vi "RelayOpen_L.vi"(0 "datain":string[](array[string])=["备注", "负载通道", "负载地址", "延时时间", "output max", "output min", "量测类型", "待测物板号"], 5 "HW CH Number":i32=4, 7 "Setup":string) -> (4 "REPORT INDECATE":string[][](array[string])=[["微安测试", "", "", "", ""], ["微安量测", "4", "0.000", "0.1", "NG"], ["微安量测", "4", "0.000", "0.1", "NG"], ["微安量测", "4", "0.000", "0.1", "NG"], ["微安量测", "4", "0.000", "0.1", "NG"]], 6 "ROW HEAD":string[](array[string]), 8 "PF":string[](array[string]), 10 "testData":string[](array[string]), 14 "数组":bool[](array[boolean]), 15 "Array":string[](array[string]))   [LabVIEW 2018]
uses:
  Subvi/Global.vi
panel:
  out "数组 2":string[](array[string])
  out "CMD 2":string
  out "测试板数":i32=4
  # "Ext.Name =Cylinder_Open;\nAddress =0;\nDelay Time =100;\nMAX.Spec =*;\nMin.Spec =*;\nTest Type =4;\nRelayH_8Bit =3,0,0,;\nRelayL_8Bit =3,0,0,;\nStandby Application =;\nStart board number =1;#"
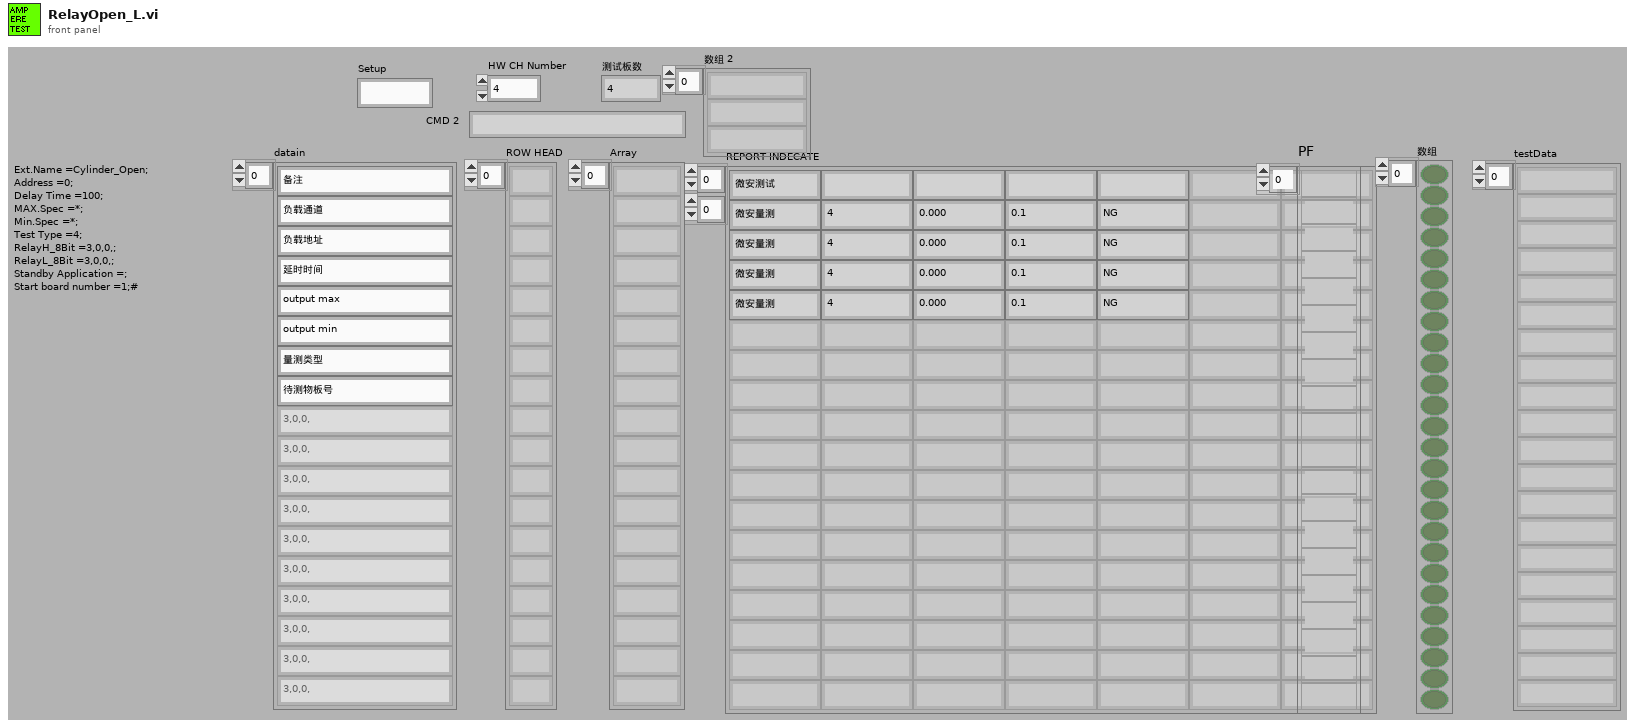
[diagram p1: front panel]
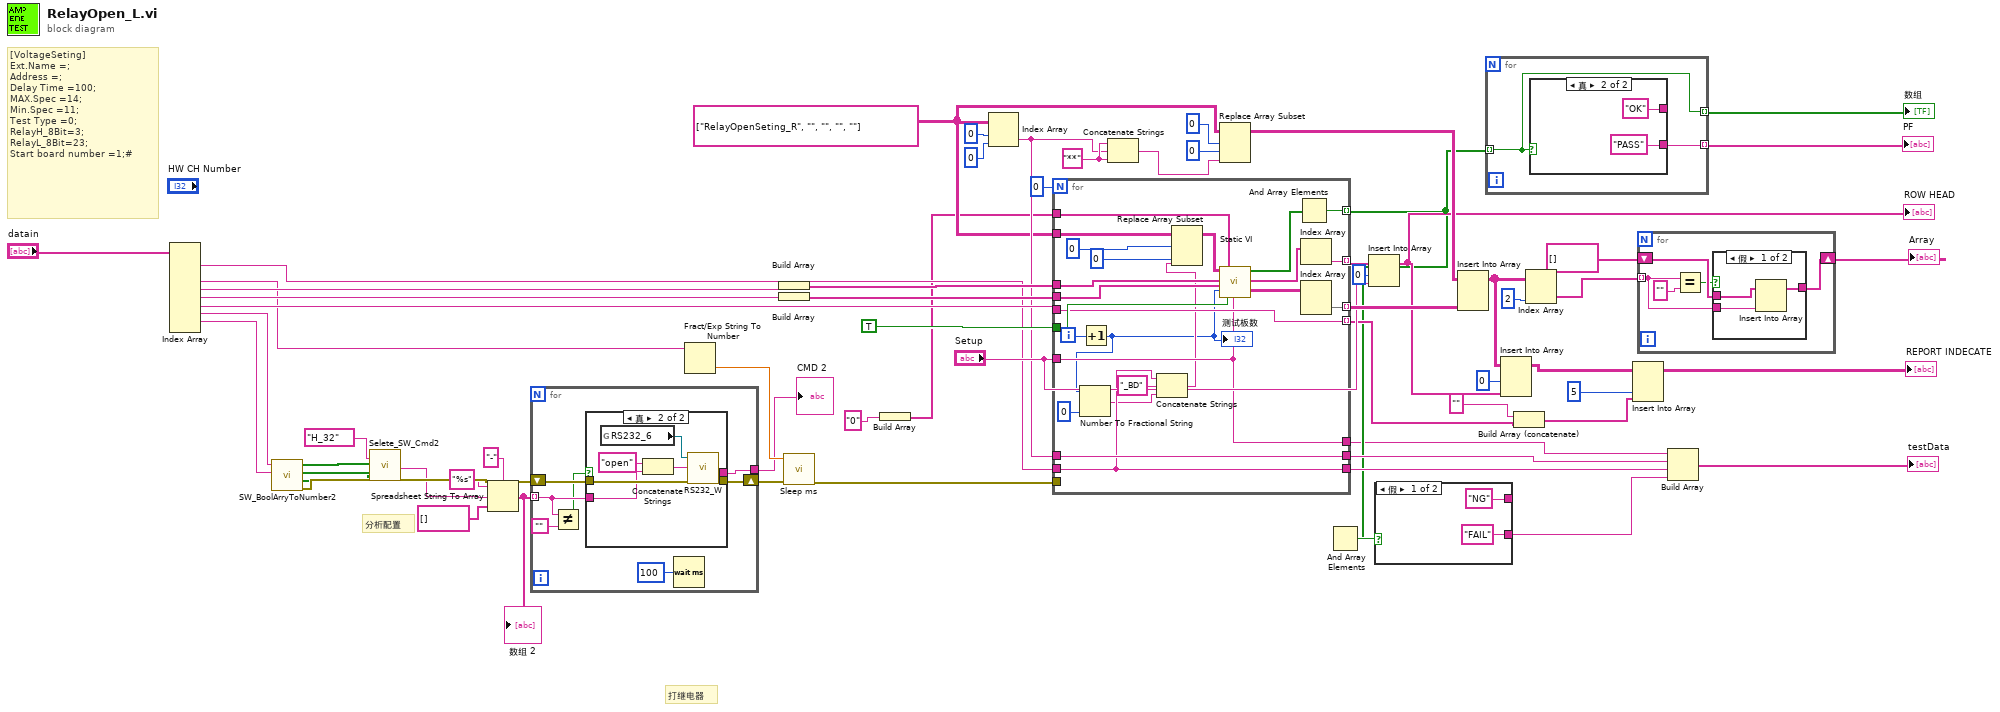
[diagram p0: block diagram]
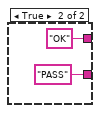
[diagram p3: hidden frame]
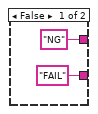
[diagram p4: hidden frame]
diagram:
  w22 = string[][] [["RelayOpenSeting_R", "", "", "", ""]]
  w56 = "**" ("字符串")
  # "分析配置"
  # "打继电器"
  # "[VoltageSeting]\nExt.Name =;\nAddress =;\nDelay Time =100;\nMAX.Spec =14;\nMin.Spec =11;\nTest Type =0;\nRelayH_8Bit=3;\nRelayL_8Bit=23;\nStart board number =1;#"
  n1 = Index Array(array="datain") -> (element #1=w23:string, element #3=w16:string, element #4=w52:string, element #5=w51:string, element #6=w39:string, element #7=w15:string, element #8=w14:string)  [unwired: 9 in, 2 out]
  n2 = call "SW_BoolArryToNumber2.vi"("L32 INUPT"=w14, "H32 INUPT"=w15) -> ("error out"=w10:errorcluster, "64 SW OUT"=w7:bool[], "L_32"=w12:bool[], "H_32"=w18:bool[])  [unwired: 6 in]
  n3 = call "Selete_SW_Cmd2.vi"("组合框"="H_32", "H_32"=w18, "L_32"=w12, "64 SW OUT"=w7, "error in (no error)"=w10) -> ("OpenStr2"=w1:string, "error out"=w9:errorcluster)  [unwired: 11 in, 2 out]
  n4 = Spreadsheet String To Array(delimiter (Tab)="-" ("分隔符(Tab)"), format string="%s" ("格式字符串"), spreadsheet string=w1, array type (2D Dbl)=string[] []) -> (array=w2:string[])
  "数组 2" <- w2
  n5 = for {
    tunnel: [w69] -> w6
    shift-right: [w70] -> w8
    shift-left: w9 -> [w71]
    tunnel: w2 -> [w67] mode=indexing
    n6 = Not Equal?(x=w67, y="") -> (x != y?=w66:bool)
    n7 = case shown="真" w66 {
      tunnel: w71 -> [w72 w79]
      tunnel: [w72 w78] -> w70
      tunnel: [_ w76] -> w69
      tunnel: w67 -> [_ w73]
      frame False {
      }
      frame True {
        n8 = global read "Global.vi" "RS232_6"() -> (w77:refnum<visa-resource-name>)
        n9 = Concatenate Strings("open", w73) -> (w75:string)
        n10 = call "RS232_W.vi"("error in (no error)"=w79, "CMD"=w75, "VISA资源名称"=w77) -> ("error out"=w78:errorcluster, "CMD 2"=w76:string)  [unwired: 6 in, 1 out]
      }
    }
    n11 = Wait (ms)(milliseconds to wait=u32 100 ("等待时间（毫秒）")) -> ()  [unwired: 1 out]
  }
  "CMD 2" <- w6
  n12 = Fract/Exp String To Number(string=w16) -> (number=w17:dbl)  [unwired: 3 in, 1 out]
  n13 = Build Array(w52) -> (w50:string[])
  n14 = Build Array(w51) -> (w49:string[])
  n15 = call "Sleep ms.vi"("error in (no error)"=w8, "等待时间（毫秒）"=w17) -> ("error out"=w13:errorcluster)  [unwired: 9 in]
  n16 = Build Array("0") -> (w19:string[])
  n17 = Index Array(array=w22, index (row)=0 ("索引 (行)"), index (col)=0 ("禁用的索引 (列)")) -> (element=w32:string)
  n18 = for {
    N: 0 -> [_]
    tunnel: w19 -> [w103]
    tunnel: w50 -> [w102]
    tunnel: w49 -> [w101]
    tunnel: "Setup" -> [w91]
    tunnel: TRUE -> [w99]
    tunnel: [w98] -> w28 mode=indexing
    tunnel: [w96] -> w45 mode=indexing
    tunnel: [w94] -> w46 mode=indexing
    tunnel: w39 -> [w93]
    tunnel: [w93] -> w35 mode=indexing
    tunnel: w32 -> [w92]
    tunnel: [w92] -> w31
    tunnel: w23 -> [w83]
    tunnel: [w83] -> w30
    tunnel: [w91] -> w25
    tunnel: w22 -> [w89]
    tunnel: w13 -> [_]
    i -> [w86]
    n19 = Increment(x=w86) -> (x+1=w80:i32)
    "测试板数" <- w80
    n20 = Number To Fractional String(number=w80, precision (6)=i16 0 ("精度(6)")) -> (F-format string=w82:string)  [unwired: 2 in]
    n21 = Concatenate Strings(w83, "_BD" ("字符串"), w82) -> (w81:string)
    n22 = Replace Array Subset(array=w89, new element=w81, index (row)=0 ("索引 (行)"), index (col)=0 ("禁用的索引 (列)")) -> (w88:string[][])
    n23 = call "Static VI.vi"("添加的数组"=w88, "Max"=w102, "Min"=w101, "板数"=w80, "INPUTSTRING"=w103, "是否为字符串对比"=w99, "SQ"=w91) -> ("P/F"=w100:bool[], "SQ out"=w97:string[], "arrauy out"=w95:string[][])  [unwired: 9 in, 1 out]
    n24 = And Array Elements(Boolean array=w100) -> (logical AND=w98:bool)
    n25 = Index Array(array=w97) -> (element=w96:string)  [unwired: 1 in]
    n26 = Index Array(array=w95) -> (element=w94:string[])  [unwired: 2 in]
  }
  n27 = Concatenate Strings(w56, w32, w56) -> (w53:string)
  n28 = Replace Array Subset(array=w22, new element=w53, index (row)=0 ("索引 (行)"), index (col)=0 ("禁用的索引 (列)")) -> (w47:string[][])
  n29 = And Array Elements(Boolean array=w28) -> (logical AND=w29:bool)
  n30 = Insert Into Array(array=w45, index=0 ("索引"), new element="Setup") -> (w41:string[])
  "ROW HEAD" <- w41
  n31 = case shown="假" w29 {
    tunnel: ["NG" "OK"] -> _
    tunnel: ["FAIL" "PASS"] -> w27
    frame False {
    }
    frame True {
    }
  }
  n32 = Insert Into Array ("数组插入")(array=w47, new element=w46) -> (w42:string[][])  [unwired: 2 in]
  n33 = for {
    tunnel: w28 -> [w108] mode=indexing
    tunnel: [w109] -> w60 mode=indexing
    tunnel: [w108] -> w24 mode=indexing
    n34 = case shown="真" w108 {
      tunnel: ["NG" "OK"] -> _
      tunnel: ["FAIL" "PASS"] -> w109
      frame False {
      }
      frame True {
      }
    }
  }
  "PF" <- w60
  "数组" <- w24
  n35 = Insert Into Array(array=w42, index (col)=0 ("禁用的索引 (列)"), new element=w41) -> (w37:string[][])  [unwired: 1 in]
  n36 = Build Array (concatenate)("" ("字符串"), w35) -> (w33:string[])
  n37 = Index Array(array=w42, index (col)=2 ("禁用的索引 (列)")) -> (element=w62:string[])  [unwired: 1 in]
  n38 = Insert Into Array(array=w37, index (col)=5 ("禁用的索引 (列)"), new element=w33) -> (→"REPORT INDECATE":string[][])  [unwired: 1 in]
  n39 = for {
    tunnel: w62 -> [w114] mode=indexing
    shift-right: [w115] -> w61
    shift-left: string[] [] ("Array") -> [w118]
    n40 = Equal?(x=w114, y="") -> (x = y?=w116:bool)
    n41 = case shown="假" w116 {
      tunnel: w118 -> [w121 w122]
      tunnel: [w120 w122] -> w115
      tunnel: w114 -> [w119 _]
      frame False {
        n42 = Insert Into Array(array=w121, new element=w119) -> (w120:string[])  [unwired: 1 in]
      }
      frame True {
      }
    }
  }
  "Array" <- w61
  n43 = Build Array(w25, w31, w30, w27) -> (→"testData":string[])
